vi "Fourier Transform (Signal to Spirograph Inputs).vi"(9 "Number of Terms":dbl, 10 "Period":dbl, 11 "Signal":cdb[](array[numeric])) -> (3 "Inputs":T1[](array[typedef]))   [LabVIEW 2020]
uses:
  Component.ctl
  <vilib>/Analysis/_algsub.llb/Real Vector Norm.vi
  <vilib>/Analysis/NI_AALPro.lvlib
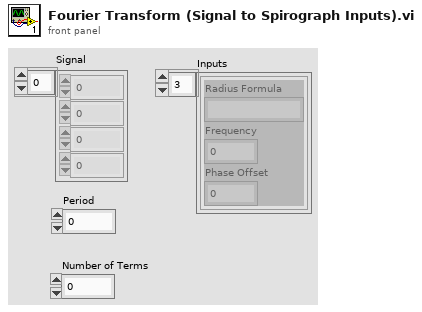
[diagram p1: front panel]
types:
  T1 = typedef "Component.ctl" = cluster{"Radius Formula":string, "Frequency":dbl, "Phase Offset":dbl}
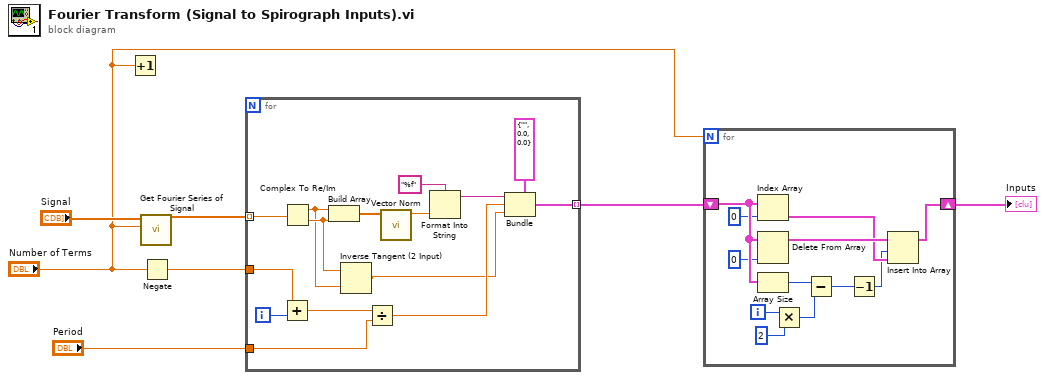
[diagram p0: block diagram]
diagram:
  n1 = Increment(x="Number of Terms") -> ()  [unwired: 1 out]
  n2 = call "Get Fourier Series of Signal.vi"("N"="Number of Terms", "Signal"="Signal") -> ("Coefficients"=w5:cdb[])  [unwired: 9 in]
  n3 = Negate(x="Number of Terms") -> (-x=w4:dbl)
  n4 = for {
    tunnel: w5 -> [w22] mode=indexing
    tunnel: [w16] -> w3 mode=indexing
    tunnel: "Period" -> [w11]
    tunnel: w4 -> [w9]
    i -> [w10]
    n5 = Add(x=w9, y=w10) -> (x+y=w8:dbl)
    n6 = Complex To Re/Im(x + iy=w22) -> (x=w13:dbl, y=w14:dbl)
    n7 = Build Array(w13, w14) -> (w21:dbl[])
    n8 = Inverse Tangent (2 Input)(1:w13, 2:w14) -> (0:w12:dbl)
    n9 = Divide(x=w8, y=w11) -> (x/y=w15:dbl)
    n10 = call-poly <vilib>:"Vector Norm.vi"("Input Vector"=w21) -> ("norm"=w20:dbl)  [unwired: 9 in, 1 out]
    n11 = Format Into String(format string="%f", w20) -> (resulting string=w18:string)  [unwired: 2 in, 1 out]
    n12 = Bundle(cluster=T1 {"Radius Formula"="", "Frequency"=0.0, "Phase Offset"=0.0}, "Radius Formula"=w18, "Frequency"=w15, "Phase Offset"=w12) -> (w16:T1)
  }
  n13 = for {
    N: "Number of Terms" -> [_]
    shift-right: [w32] -> w2
    shift-left: w3 -> [w30]
    i -> [w25]
    n14 = Index Array(array=w30, index=0) -> (element=w33:T1)
    n15 = Delete From Array(array=w30, index=0) -> (array with subset deleted=w34:T1[])  [unwired: 1 in, 1 out]
    n16 = Array Size(array=w30) -> (size(s)=w31:i32)
    n17 = Multiply(x=w25, y=2) -> (x*y=w23:i32)
    n18 = Subtract(x=w31, y=w23) -> (x-y=w29:i32)
    n19 = Decrement(x=w29) -> (x-1=w28:i32)
    n20 = Insert Into Array(array=w34, index=w28, new element=w33) -> (w32:T1[])
  }
  "Inputs" <- w2
